vi "txt-array.vi"(10 "file (use dialog)":path=path "C:/Users/Azmat/Desktop/Labview/协议.txt") -> (2 "输出数组":T1(array[cluster]))   [LabVIEW 2016]
panel:
  out "appended array":string[](array[string])
  in  "end pattern string":string="#end"
  in  "start pattern string":string="#start"
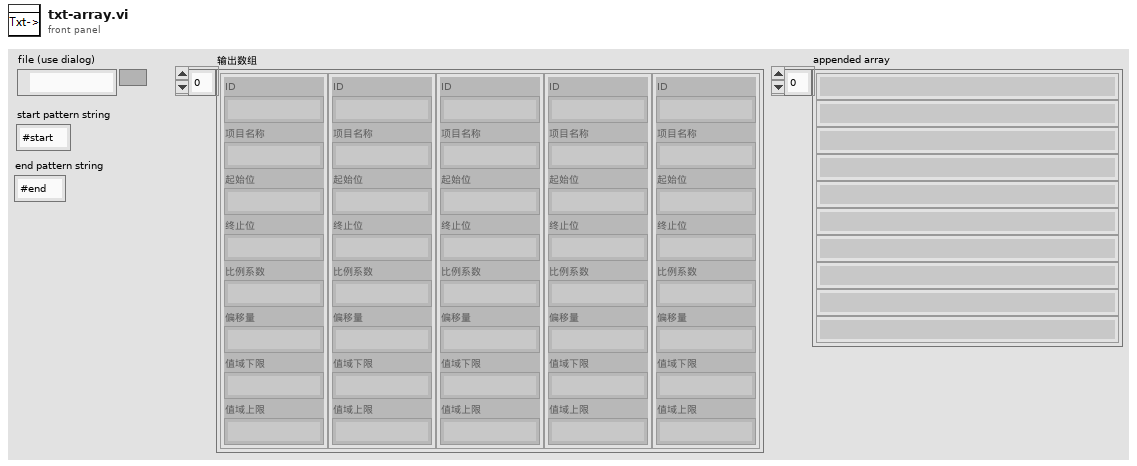
[diagram p1: front panel]
types:
  T1 = cluster{"ID":string, "项目名称":string, "起始位":string, "终止位":string, "比例系数":string, "偏移量":string, "值域下限":string, "值域上限":string}[]
  T2 = cluster{"ID":string, "项目名称":string, "起始位":string, "终止位":string, "比例系数":string, "偏移量":string, "值域上限":string, "值域下限":string}[]
  T3 = cluster{"ID":string, "项目名称":string, "起始位":string, "终止位":string, "比例系数":string, "偏移量":string, "值域上限":string, "值域下限":string}
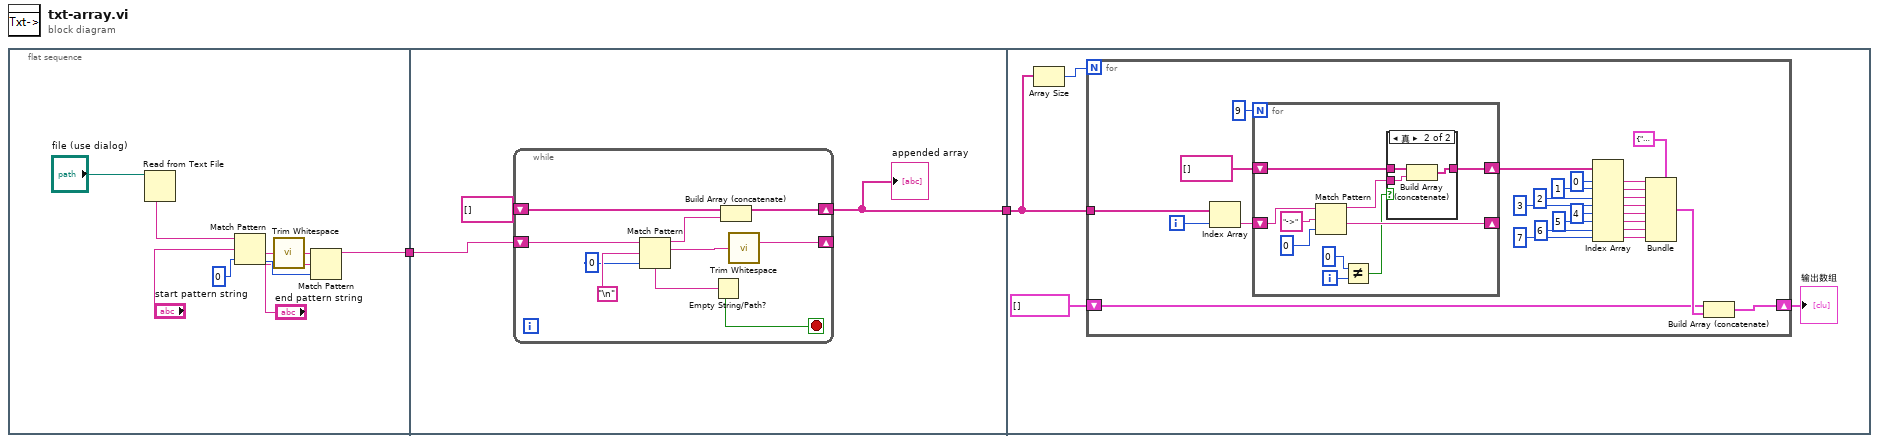
[diagram p0: block diagram]
diagram:
  n1 = flat-sequence {
    tunnel: [w3] -> w2
    tunnel: w2 -> [w13]
    tunnel: [w12] -> w1
    tunnel: w1 -> [w24]
    frame #0 {
      n2 = Read from Text File(file (use dialog)="file (use dialog)") -> (text=w10:string)  [unwired: 3 in, 3 out]
      n3 = Match Pattern(string=w10, regular expression="start pattern string", offset (0)=0) -> (after substring=w4:string, offset past match=w7:i32)  [unwired: 2 out]
      n4 = call <vilib>:"Trim Whitespace.vi"("string"=w4) -> ("trimmed string"=w5:string)  [unwired: 1 in]
      n5 = Match Pattern(string=w5, regular expression="end pattern string", offset (0)=w7) -> (before substring=w3:string)  [unwired: 3 out]
    }
    frame #1 {
      n6 = while {
        shift-right: [w20] -> w12
        shift-left: string[] [] ("appended array") -> [w21]
        shift-right: [w17] -> _
        shift-left: w13 -> [w19]
        stop <- w23 stop-if-true
        n7 = Match Pattern(string=w19, regular expression="\n", offset (0)=0) -> (before substring=w22:string, after substring=w18:string)  [unwired: 2 out]
        n8 = Empty String/Path?(string/path=w18) -> (empty?=w23:bool)
        n9 = Build Array (concatenate)(w21, w22) -> (w20:string[])
        n10 = call <vilib>:"Trim Whitespace.vi"("string"=w18) -> ("trimmed string"=w17:string)  [unwired: 1 in]
      }
      "appended array" <- w12
    }
    frame #2 {
      n11 = Array Size(array=w24) -> (size(s)=w25:i32)
      n12 = for {
        N: w25 -> [_]
        tunnel: w24 -> [w53]
        shift-right: [w31] -> w26
        shift-left: T2 [] -> [w28]
        i -> [w32]
        n13 = Index Array(array=w53, index=w32) -> (element=w51:string)
        n14 = for {
          N: 9 -> [_]
          shift-right: [w60] -> _
          shift-left: w51 -> [w61]
          shift-right: [w57] -> w49
          shift-left: string[] [] -> [w58]
          i -> [w56]
          n15 = Match Pattern(string=w61, regular expression="->", offset (0)=0) -> (before substring=w59:string, after substring=w60:string)  [unwired: 2 out]
          n16 = Not Equal?(x=0, y=w56) -> (x != y?=w54:bool)
          n17 = case shown="真" w54 {
            tunnel: w59 -> [_ w67]
            tunnel: w58 -> [w64 w66]
            tunnel: [w64 w65] -> w57
            frame False {
            }
            frame True {
              n18 = Build Array (concatenate)(w66, w67) -> (w65:string[])
            }
          }
        }
        n19 = Index Array(array=w49, index #1=0 ("index"), index #2=1 ("index"), index #3=2 ("index"), index #4=3 ("index"), index #5=4 ("index"), index #6=5 ("index"), index #7=6 ("index"), index #8=7 ("index")) -> (element #1=w48:string, element #2=w39:string, element #3=w38:string, element #4=w37:string, element #5=w36:string, element #6=w35:string, element #7=w34:string, element #8=w33:string)
        n20 = Bundle(cluster=T3 {"ID"="", "项目名称"="", "起始位"="", "终止位"="", "比例系数"="", "偏移量"="", "值域上限"="", "值域下限"=""} ("Cluster"), "ID"=w48, "项目名称"=w39, "起始位"=w38, "终止位"=w37, "比例系数"=w36, "偏移量"=w35, "值域上限"=w34, "值域下限"=w33) -> (w29:T3)
        n21 = Build Array (concatenate)(w28, w29) -> (w31:T2)
      }
      "输出数组" <- w26
    }
  }
